vi "Display.vi"(8 "error in (no error)":errorcluster, 11 "ADDI-Data in":refnum<class "ADDI-Data.lvclass">) -> (0 "error out":errorcluster, 3 "ADDI-Data out":refnum<class "ADDI-Data.lvclass">)   [LabVIEW 2014, in "ADDI-Data.lvlib" / "ADDI-Data.lvclass"]
uses:
  ADDI-Data.lvclass
panel:
  in  "STOP":bool
  out "Entradas Digitales":bool[](array[boolean])
  out "Encoder":dbl(knob) scale=0.0..360.0
  out "Entrada Analogica":dbl(graph)
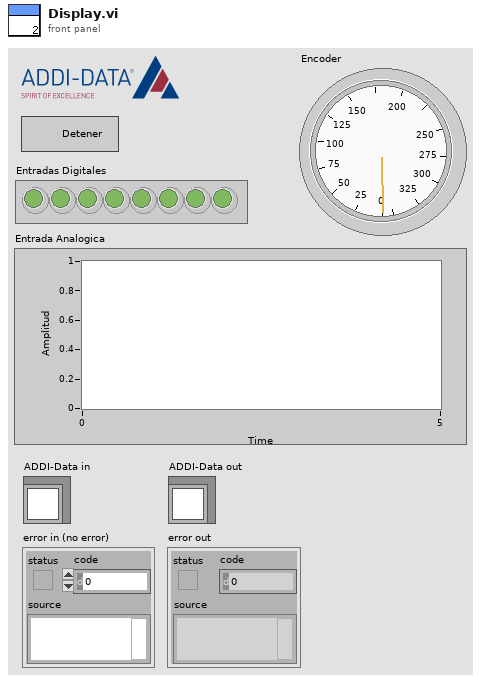
[diagram p1: front panel]
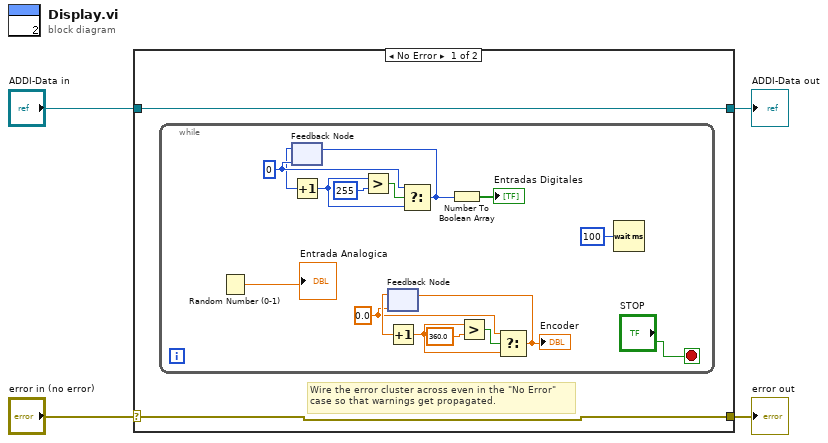
[diagram p0: block diagram]
diagram:
  n1 = case shown="No Error" "error in (no error)" {
    selector: "error in (no error)" -> [w5 w24]
    tunnel: [w5 w24] -> w3
    tunnel: [w6 w23] -> w1
    tunnel: "ADDI-Data in" -> [w6 w23]
    frame No Error {
      # "Wire the error cluster across even in the \"No Error\"\ncase so that warnings get propagated."
      n2 = while {
        stop <- "STOP" stop-if-true
        w15 = u8 0
        w16 = 0.0
        n3 = Random Number (0-1)() -> (number: 0 to 1=→"Entrada Analogica":dbl)
        n4 = feedback #1(w15) -> (w11:u8)
        n5 = Increment(x=w11) -> (x+1=w14:u8)
        n6 = Greater?(x=w14, y=u8 255) -> (0:w13:bool)
        n7 = feedback #2(w16) -> (w21:dbl)
        n8 = Increment(x=w21) -> (x+1=w18:dbl)
        n9 = Select(t=w15, s=w13, f=w14) -> (s? t:f=w10:u8)
        n10 = feedback-in #1(w10) -> ()
        n11 = Number To Boolean Array(number=w10) -> (Boolean array=→"Entradas Digitales":bool[])
        n12 = Greater?(x=w18, y=360.0) -> (0:w19:bool)
        n13 = Select(t=w16, s=w19, f=w18) -> (s? t:f=w17:dbl)
        "Encoder" <- w17
        n14 = feedback-in #2(w17) -> ()
        n15 = Wait (ms)(milliseconds to wait=u32 100) -> ()  [unwired: 1 out]
      }
    }
    frame Error {
    }
  }
  "error out" <- w3
  "ADDI-Data out" <- w1
